vi "Read tcp connection.vi"(8 "error in (no error)":errorcluster, 11 "TCP Interface in":refnum<class "TCP Interface.lvclass">) -> (0 "error out":errorcluster, 2 "tcp connection":refnum<k5>, 3 "TCP Interface out":refnum<class "TCP Interface.lvclass">)   [LabVIEW 2021, in "TCP Interface.lvclass"]
uses:
  TCP Interface.lvclass
  TCP Interface.lvclass/TCP Interface.ctl
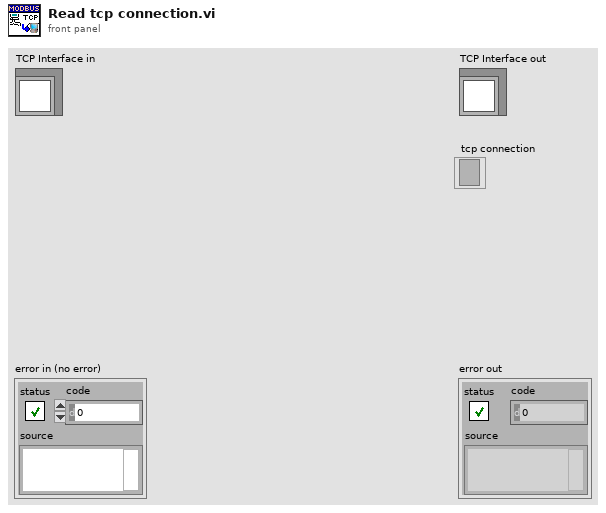
[diagram p1: front panel]
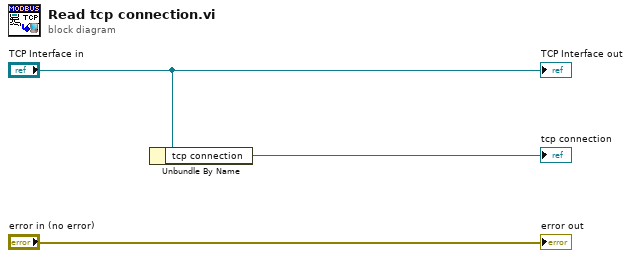
[diagram p0: block diagram]
diagram:
  n1 = Unbundle By Name("TCP Interface in") -> ("tcp connection"=→"tcp connection":refnum<k5>)
  "error out" <- "error in (no error)"
  "TCP Interface out" <- "TCP Interface in"
